vi "Silent Main.vi"   [LabVIEW 2020]
types:
  T1 = enum32{"Invalid", "Standard", "Closed", "Hidden", "Minimized", "Maximized"}
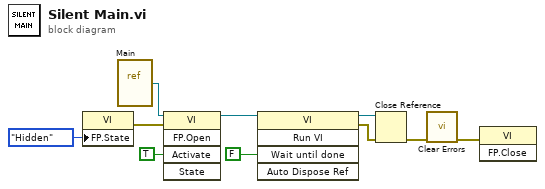
[diagram p0: block diagram]
diagram:
  n1 = property class="VI"("FP.State"=T1."Hidden" ("Front Panel Window:State")) -> (error out=w9:errorcluster)  [unwired: 2 in, 1 out]
  n2 = vi-ref "Main.vi"() -> (w4:refnum<vi>)
  n3 = invoke class="VI" method="FP.Open"(reference=w4, error in=w9, "Activate"=TRUE ("Activate?")) -> (reference out=w3:refnum<vi>)  [unwired: 2 in, 4 out]
  n4 = invoke class="VI" method="Run VI"(reference=w3, "Wait until done"=FALSE ("Wait Until Done")) -> (reference out=w5:refnum<vi>, error out=w10:errorcluster)  [unwired: 3 in, 3 out]
  n5 = Close Reference(reference=w5, error in (no error)=w10) -> (error out=w8:errorcluster)
  n6 = call <vilib>:"Clear Errors.vi"("error in (no error)"=w8) -> ("error out"=w7:errorcluster)  [unwired: 5 in, 1 out]
  n7 = invoke class="VI" method="FP.Close"(error in=w7) -> ()  [unwired: 2 in, 3 out]
